vi "Immediate Data Log Trigger.vi"(8 "error in (no error)":errorcluster {"code" format="%.0x"}, 11 "VISA resource name":refnum<visa-resource-name>) -> (0 "error out":errorcluster {"code" format="%.0x"}, 3 "VISA resource name out":refnum<visa-resource-name>)   [LabVIEW 2014, in "Agilent N6700 Series.lvlib"]
doc: "Sends an immediate trigger signal to the data logger. This will trigger the data log regardless of the selected trigger source.\n\n<b>Notes:</b>\n(1) The data logger must be initiated before triggered.\n(2) This VI only applies to the N6705B and N6705C DC Power Analyzer."
uses:
  Agilent N6700 Series.lvlib
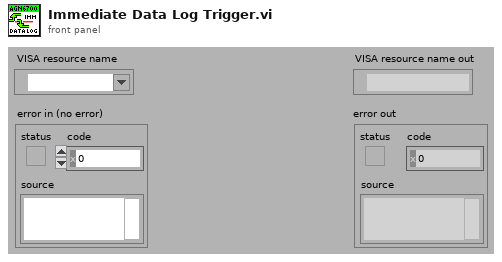
[diagram p1: front panel]
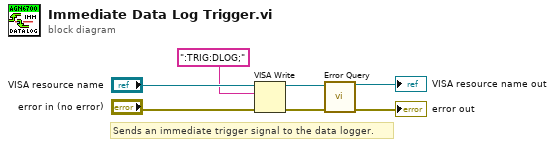
[diagram p0: block diagram]
diagram:
  # "Sends an immediate trigger signal to the data logger."
  n1 = VISA Write(VISA resource name="VISA resource name", write buffer=":TRIG:DLOG;", error in (no error)="error in (no error)") -> (VISA resource name out=w3:refnum<visa-resource-name>, error out=w2:errorcluster)  [unwired: 1 out]
  n2 = call "Error Query.vi"("VISA resource name"=w3, "error in (no error)"=w2) -> ("VISA resource name out"=→"VISA resource name out":refnum<visa-resource-name>, "error out"=→"error out":errorcluster)  [unwired: 10 in, 2 out]
